vi "Config BERT Input.vi"(0 "VISA Resource Name":refnum<visa-resource-name>, 1 "Clock Gate (F:OFF)":bool, 2 "Clock Gate Polarity (T:POS)":bool=TRUE, 5 "Clock Polarity (T:POSITIVE)":bool=TRUE, 7 "Data Polarity (T:POSITIVE)":bool=TRUE, 9 "Impedance (F:TTL)":bool, 11 "error in (no error)":errorcluster {"code" format="%.0x"}) -> (4 "VISA Resource Name Out":refnum<visa-resource-name>, 15 "error out":errorcluster {"code" format="%.0x"})   [LabVIEW 2014, in "Agilent ESG Series.lvlib"]
doc: "This VI is used to configure the parameters associated with the input connectors for the bit error rate tests."
uses:
  Agilent ESG Series.lvlib
panel:
  # "POSITIVE"
  # "NEGATIVE"
  # "POSITIVE"
  # "NEGATIVE"
  # "ON"
  # "OFF"
  # "POSITIVE"
  # "NEGATIVE"
  # "75 OHM"
  # "TTL"
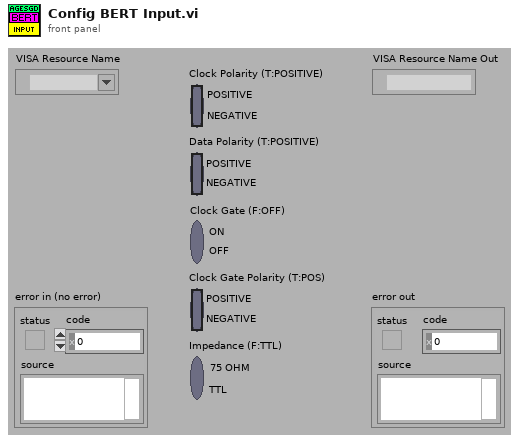
[diagram p1: front panel]
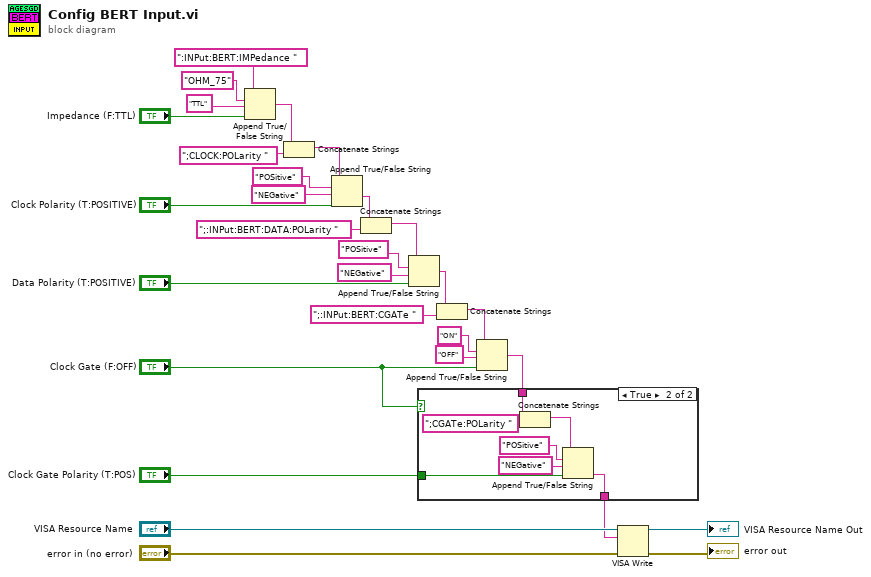
[diagram p0: block diagram]
diagram:
  n1 = Append True/False String(1:"Impedance (F:TTL)", 2:"TTL" ("false string"), 3:"OHM_75" ("true string"), 4:":INPut:BERT:IMPedance " ("string (\"\")")) -> (0:w4:string)
  n2 = Concatenate Strings(w4, ";CLOCK:POLarity " ("string (\"\")")) -> (w2:string)
  n3 = Append True/False String(1:"Clock Polarity (T:POSITIVE)", 2:"NEGative" ("false string"), 3:"POSitive" ("true string"), 4:w2) -> (0:w23:string)
  n4 = Concatenate Strings(w23, ";:INPut:BERT:DATA:POLarity ") -> (w19:string)
  n5 = Append True/False String(1:"Data Polarity (T:POSITIVE)", 2:"NEGative" ("false string"), 3:"POSitive" ("true string"), 4:w19) -> (0:w14:string)
  n6 = Concatenate Strings(w14, ";:INPut:BERT:CGATe ") -> (w15:string)
  n7 = Append True/False String(1:"Clock Gate (F:OFF)", 2:"OFF" ("false string"), 3:"ON" ("true string"), 4:w15) -> (0:w13:string)
  n8 = case shown="True" "Clock Gate (F:OFF)" {
    tunnel: w13 -> [w30 w33]
    tunnel: "Clock Gate Polarity (T:POS)" -> [_ w32]
    tunnel: [w30 w31] -> w1
    frame False {
    }
    frame True {
      n9 = Concatenate Strings(w33, ";CGATe:POLarity ") -> (w34:string)
      n10 = Append True/False String(1:w32, 2:"NEGative" ("false string"), 3:"POSitive" ("true string"), 4:w34) -> (0:w31:string)
    }
  }
  n11 = VISA Write(VISA resource name="VISA Resource Name", write buffer=w1, error in (no error)="error in (no error)") -> (VISA resource name out=→"VISA Resource Name Out":refnum<visa-resource-name>, error out=→"error out":errorcluster)  [unwired: 1 out]
